vi "SaveDataQDCV965A.vi"(0 "String":string, 1 "Save Data?":bool, 5 "File Handle":T1 format="%.0x", 9 "Buff":u32[](array[numeric]), 11 "error in (no error)":errorcluster, 12 "Module":string="QDC Data") -> (4 "# Events Acquired (VME)":u32, 15 "error out":errorcluster)   [LabVIEW 2014]
uses:
  <vilib>/addons/h5labview2/base/hid_t.ctl
  <vilib>/addons/h5labview2/base/lib_path.vi
  <vilib>/addons/h5labview2/base/H5Equery.vi
  <vilib>/addons/h5labview2/dataset/H5Dwrite.llb/H5Dwrite.xnode
  <vilib>/addons/h5labview2/group/H5G.lvlib
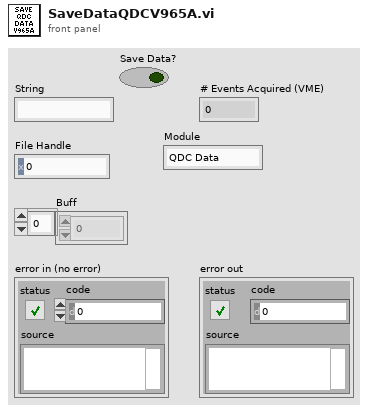
[diagram p1: front panel]
types:
  T1 = typedef "hid_t.ctl" = i32
  T2 = typedef "QDCDataCluster.ctl" = cluster{"Channel":u8, "QDC Data":sgl, "LowRange?":bool, "Overflow?":bool}
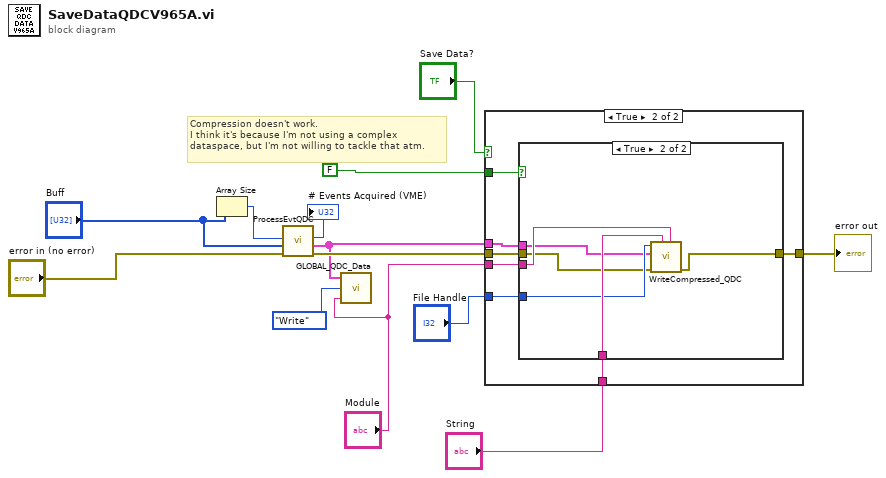
[diagram p0: block diagram]
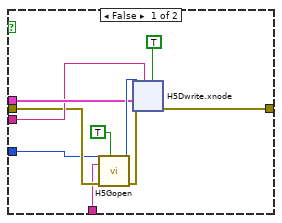
[diagram p3: hidden frame]
diagram:
  # "Compression doesn't work.\nI think it's because I'm not using a complex\ndataspace, but I'm not willing to tackle that atm."
  n1 = Array Size(array="Buff") -> (size(s)=w10:i32)
  n2 = call "ProcessEvtQDC.vi"("error in"="error in (no error)", "Encoded Data"="Buff", "# data points in evt"=w10) -> ("error out"=w12:errorcluster, "Decoded Data"=w2:T2[], "# Events"=→"# Events Acquired (VME)":u32)  [unwired: 6 in]
  n3 = call "GLOBAL_QDC_Data.vi"("Module"="Module", "State"=enum16{"Initialise", "Write", "Read"}."Write", "Input Data"=w2) -> ()  [unwired: 1 in, 2 out]
  n4 = case shown="True" "Save Data?" {
    tunnel: [w14 w21] -> w13
    tunnel: w12 -> [w14 w18]
    tunnel: w2 -> [_ w20]
    tunnel: "Module" -> [_ w19]
    tunnel: "File Handle" -> [_ w17]
    tunnel: "String" -> [_ w16]
    tunnel: FALSE ("Compress?") -> [_ w15]
    frame False {
    }
    frame True {
      n5 = case shown="True" w15 {
        tunnel: [w30 w50] -> w21
        tunnel: w20 -> [w29 w52]
        tunnel: w19 -> [w28 w55]
        tunnel: w18 -> [w25 w51]
        tunnel: w17 -> [w23 w53]
        tunnel: w16 -> [w22 w54]
        frame False {
          n6 = call <vilib>:"H5Gopen.vi"("create? (F)"=TRUE, "error in (no error)"=w25, "name"=w22, "ref in"=w23) -> ("error out"=w24:errorcluster, "group out"=w31:T1)  [unwired: 6 in]
          n7 = xnode "H5Dwrite.xnode"("replace? (F)"=TRUE, "dataset name"=w28, "error in (no error)"=w24, "data"=w29, "ref in"=w31) -> ("error out"=w30:errorcluster)  [unwired: 2 in, 2 out]
        }
        frame True {
          n8 = call "WriteCompressed_QDC.vi"("Module"=w55, "name"=w54, "error in"=w51, "Decoded Data"=w52, "File Handle"=w53) -> ("error out"=w50:errorcluster)  [unwired: 6 in]
        }
      }
    }
  }
  "error out" <- w13
